vi "Test Errors Are Cleared.vi"(8 "error in (no error)":errorcluster, 11 "Test Case In":refnum<class "Error Handler Tests.lvclass">) -> (0 "error out":errorcluster, 3 "Test Case Out":refnum<class "Error Handler Tests.lvclass">)   [LabVIEW 2020, in "Error Handler Tests.lvclass"]
uses:
  Error Handler Tests.lvclass
  C:/Program Files (x86)/National Instruments/LabVIEW 2020/vi.lib/Astemes/LUnit/Test Case.lvclass
  <vilib>/Astemes/LUnit/Test Case.lvclass/Test Case.ctl
  <vilib>/Astemes/LUnit/Palette/Pass.vi
  <vilib>/Astemes/LUnit/Palette/Fail.vi
  <vilib>/Astemes/LUnit/Set Assertion Type.vi
  <vilib>/Astemes/LUnit/Add test result.vi
  <vilib>/Astemes/LUnit/LUnit Record Assertion Result.vi
  <vilib>/Astemes/LUnit/LUnit Aggregate Assertion Results.vi
  <vilib>/Astemes/LUnit/Method Result/LUnit Merge Status.vi
  <vilib>/Astemes/LUnit/LUnit Concatenate result strings.vi
  source/User Interface/Error Handler/Error Handler.lvclass
  <vilib>/Astemes/LUnit/Test Case.lvclass
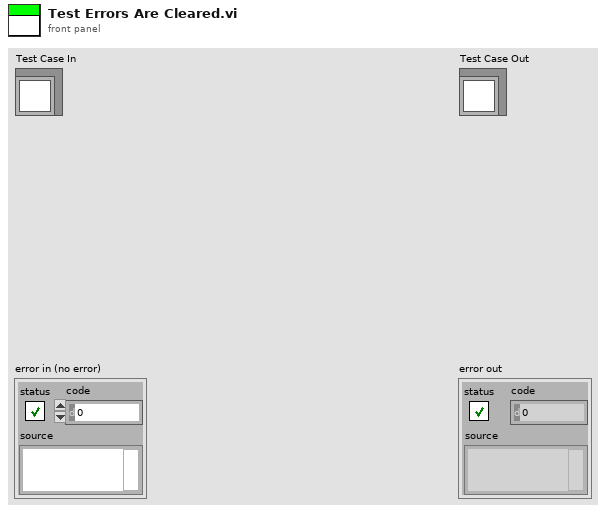
[diagram p1: front panel]
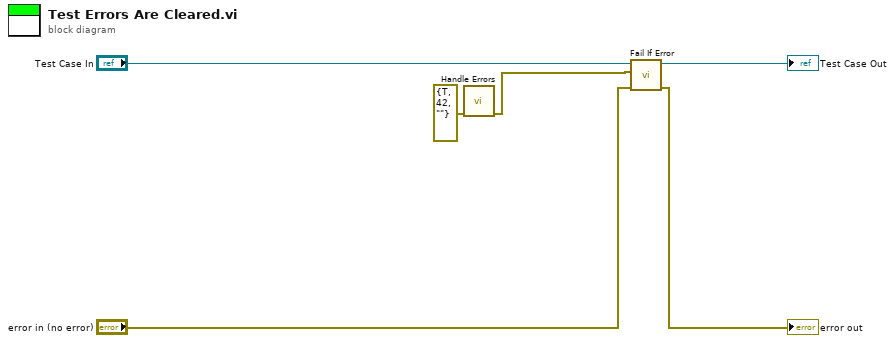
[diagram p0: block diagram]
diagram:
  n1 = call "Handle Errors.vi"("error in (no error)"=errorcluster {"status"=TRUE, "code"=42, "source"=""}) -> ("error out"=w2:errorcluster)  [unwired: 10 in]
  n2 = call <vilib>:"Fail If Error.vi"("error in (no error)"="error in (no error)", "Assert error"=w2, "LUnit Test Case In"="Test Case In") -> ("error out"=→"error out":errorcluster, "LUnit Test Case Out"=→"Test Case Out":refnum<class "Error Handler Tests.lvclass">)  [unwired: 7 in]
